vi "DataSenalesDTMF.vi"() -> (0 "Data_Senales_DTMF":T1(array[cluster])=[{"Frecuencia_Alta"=1209.0, "Frecuencia_Baja"=697.0, "Indicador_Tecla"=1.0, "Tecla"="1"}, {"Frecuencia_Alta"=1336.0, "Frecuencia_Baja"=697.0, "Indicador_Tecla"=2.0, "Tecla"="2"}, {"Frecuencia_Alta"=1477.0, "Frecuencia_Baja"=697.0, "Indicador_Tecla"=3.0, "Tecla"="3"}, {"Frecuencia_Alta"=1633.0, "Frecuencia_Baja"=697.0, "Indicador_Tecla"=12.0, "Tecla"="A"}, {"Frecuencia_Alta"=1209.0, "Frecuencia_Baja"=770.0, "Indicador_Tecla"=4.0, "Tecla"="4"}, {"Frecuencia_Alta"=1336.0, "Frecuencia_Baja"=770.0, "Indicador_Tecla"=5.0, "Tecla"="5"}, {"Frecuencia_Alta"=1477.0, "Frecuencia_Baja"=770.0, "Indicador_Tecla"=6.0, "Tecla"="6"}, {"Frecuencia_Alta"=1633.0, "Frecuencia_Baja"=770.0, "Indicador_Tecla"=13.0, "Tecla"="B"}, {"Frecuencia_Alta"=1209.0, "Frecuencia_Baja"=852.0, "Indicador_Tecla"=7.0, "Tecla"="7"}, {"Frecuencia_Alta"=1336.0, "Frecuencia_Baja"=852.0, "Indicador_Tecla"=8.0, "Tecla"="8"}, {"Frecuencia_Alta"=1477.0, "Frecuencia_Baja"=852.0, "Indicador_Tecla"=9.0, "Tecla"="9"}, {"Frecuencia_Alta"=1633.0, "Frecuencia_Baja"=852.0, "Indicador_Tecla"=14.0, "Tecla"="C"}, {"Frecuencia_Alta"=1209.0, "Frecuencia_Baja"=941.0, "Indicador_Tecla"=10.0, "Tecla"="*"}, {"Frecuencia_Alta"=1336.0, "Frecuencia_Baja"=941.0, "Indicador_Tecla"=0.0, "Tecla"="0"}, {"Frecuencia_Alta"=1477.0, "Frecuencia_Baja"=941.0, "Indicador_Tecla"=11.0, "Tecla"="#"}, {"Frecuencia_Alta"=1633.0, "Frecuencia_Baja"=941.0, "Indicador_Tecla"=15.0, "Tecla"="D"}])   [LabVIEW 2018]
panel:
  in  "Data_Senales_DTMF_Control":T1(array[cluster])=[{"Frecuencia_Alta"=1209.0, "Frecuencia_Baja"=697.0, "Indicador_Tecla"=1.0, "Tecla"="1"}, {"Frecuencia_Alta"=1336.0, "Frecuencia_Baja"=697.0, "Indicador_Tecla"=2.0, "Tecla"="2"}, {"Frecuencia_Alta"=1477.0, "Frecuencia_Baja"=697.0, "Indicador_Tecla"=3.0, "Tecla"="3"}, {"Frecuencia_Alta"=1633.0, "Frecuencia_Baja"=697.0, "Indicador_Tecla"=12.0, "Tecla"="A"}, {"Frecuencia_Alta"=1209.0, "Frecuencia_Baja"=770.0, "Indicador_Tecla"=4.0, "Tecla"="4"}, {"Frecuencia_Alta"=1336.0, "Frecuencia_Baja"=770.0, "Indicador_Tecla"=5.0, "Tecla"="5"}, {"Frecuencia_Alta"=1477.0, "Frecuencia_Baja"=770.0, "Indicador_Tecla"=6.0, "Tecla"="6"}, {"Frecuencia_Alta"=1633.0, "Frecuencia_Baja"=770.0, "Indicador_Tecla"=13.0, "Tecla"="B"}, {"Frecuencia_Alta"=1209.0, "Frecuencia_Baja"=852.0, "Indicador_Tecla"=7.0, "Tecla"="7"}, {"Frecuencia_Alta"=1336.0, "Frecuencia_Baja"=852.0, "Indicador_Tecla"=8.0, "Tecla"="8"}, {"Frecuencia_Alta"=1477.0, "Frecuencia_Baja"=852.0, "Indicador_Tecla"=9.0, "Tecla"="9"}, {"Frecuencia_Alta"=1633.0, "Frecuencia_Baja"=852.0, "Indicador_Tecla"=14.0, "Tecla"="C"}, {"Frecuencia_Alta"=1209.0, "Frecuencia_Baja"=941.0, "Indicador_Tecla"=10.0, "Tecla"="*"}, {"Frecuencia_Alta"=1336.0, "Frecuencia_Baja"=941.0, "Indicador_Tecla"=0.0, "Tecla"="0"}, {"Frecuencia_Alta"=1477.0, "Frecuencia_Baja"=941.0, "Indicador_Tecla"=11.0, "Tecla"="#"}, {"Frecuencia_Alta"=1633.0, "Frecuencia_Baja"=941.0, "Indicador_Tecla"=15.0, "Tecla"="D"}]
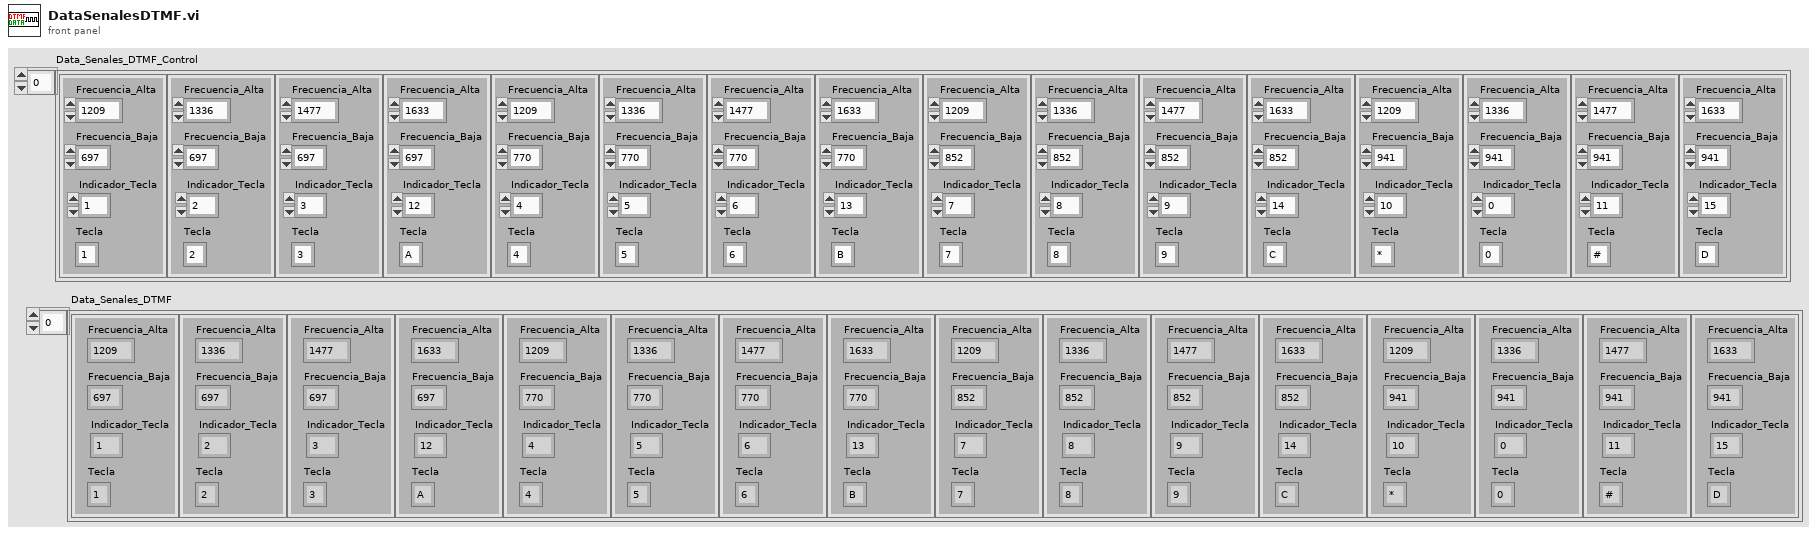
[diagram p1: front panel]
types:
  T1 = cluster{"Frecuencia_Alta":dbl, "Frecuencia_Baja":dbl, "Indicador_Tecla":dbl, "Tecla":string}[]
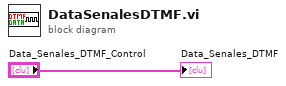
[diagram p0: block diagram]
diagram:
  "Data_Senales_DTMF" <- "Data_Senales_DTMF_Control"
